vi "set_params.vi"(0 "smc100 in":refnum<class "smc100.lvclass">, 3 "error in (no error)":errorcluster) -> (7 "smc100 out":refnum<class "smc100.lvclass">, 10 "error out":errorcluster)   [LabVIEW 2019, in "smc100.lvlib" / "smc100.lvclass"]
uses:
  smc100.lvclass
  smc100.lvclass/smc100.ctl
  Write COM port.vi
panel:
  in  "OK Button":bool
  in  "COM port":u8=3
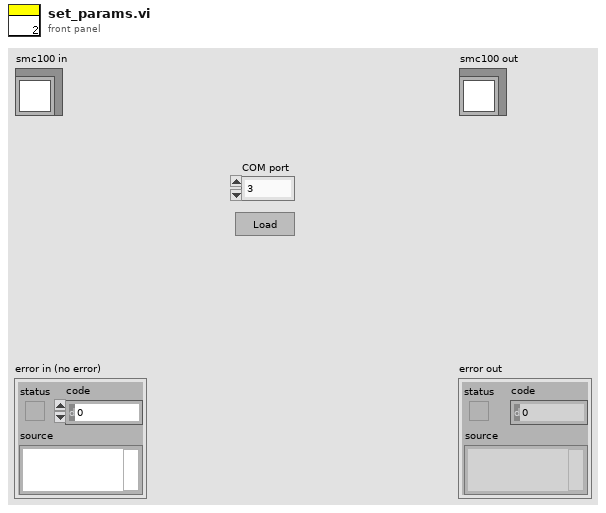
[diagram p1: front panel]
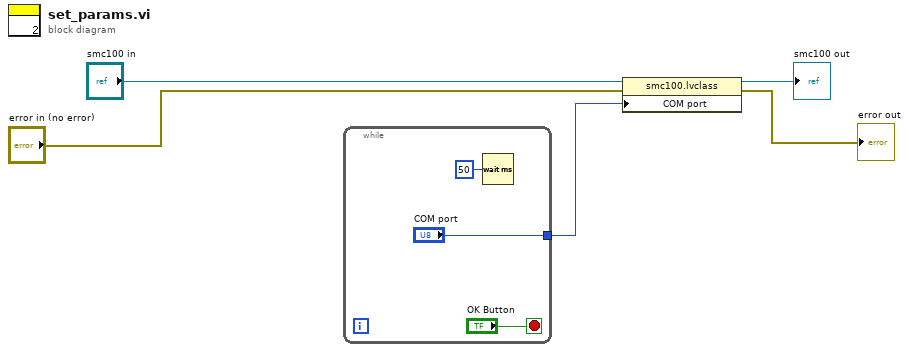
[diagram p0: block diagram]
diagram:
  n1 = while {
    tunnel: ["COM port"] -> w1
    stop <- "OK Button" stop-if-true
    n2 = Wait (ms)(milliseconds to wait=u32 50) -> ()  [unwired: 1 out]
  }
  n3 = property class="smc100.lvclass"(reference="smc100 in", error in="error in (no error)", "COM port"=w1) -> (reference out=→"smc100 out":refnum<class "smc100.lvclass">, error out=→"error out":errorcluster)
